vi "GetFieldsFromCoeffsFile_v1.vi"(11 "all rows":dbl[][](array[numeric])) -> (3 "Array":string[](array[string]))   [LabVIEW 2023]
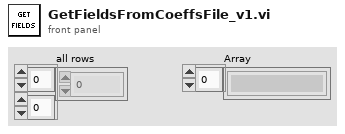
[diagram p1: front panel]
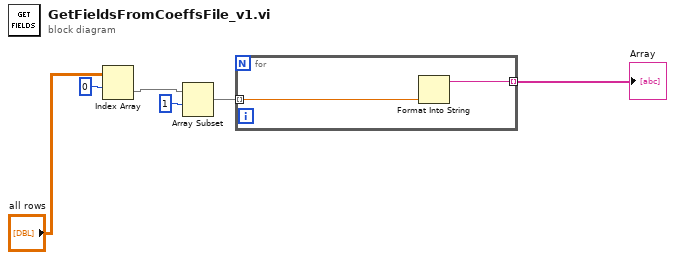
[diagram p0: block diagram]
diagram:
  n1 = Index Array(array="all rows", index (row)=0) -> (element=w3:dbl[])  [unwired: 1 in]
  n2 = Array Subset(array=w3, index=1) -> (w4:dbl[])  [unwired: 1 in]
  n3 = for {
    tunnel: w4 -> [w8] mode=indexing
    tunnel: [w7] -> w5 mode=indexing
    n4 = Format Into String(w8) -> (resulting string=w7:string)  [unwired: 3 in, 1 out]
  }
  "Array" <- w5
